vi "niFpgaHandshakePaletteMethodNodeMergeVi.vi"   [LabVIEW 2017]
doc: "Invokes a method on a handshake item on the FPGA."
uses:
  <vilib>/rvi/DataTransferAndStorage/Container/XNode/niFpgaContainer.xnode
  <vilib>/rvi/DataTransferAndStorage/Handshake/Emulation/niFpgaHandshakeEmulation.vi
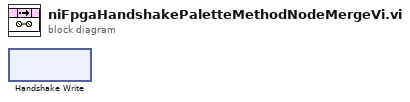
[diagram p0: block diagram]
diagram:
  n1 = xnode "Handshake Write"() -> ()  [unwired: 1 in, 1 out]
